vi "Read Monitor Data.vi"(8 "error in (no error)":errorcluster, 11 "Actor Monitor New in":refnum<class "Actor Monitor.lvclass">) -> (0 "error out":errorcluster, 2 "Monitored Actor.lvlib:Monitor Data.lvclass":refnum<class "Monitor Data.lvclass">, 3 "Actor Monitor New out":refnum<class "Actor Monitor.lvclass">)   [LabVIEW 2023, in "Monitored Actor.lvlib" / "Actor Monitor.lvclass"]
uses:
  Actor Monitor.lvclass
  Monitor Data/Monitor Data.lvclass
  Actor Monitor.lvclass/Actor Monitor.ctl
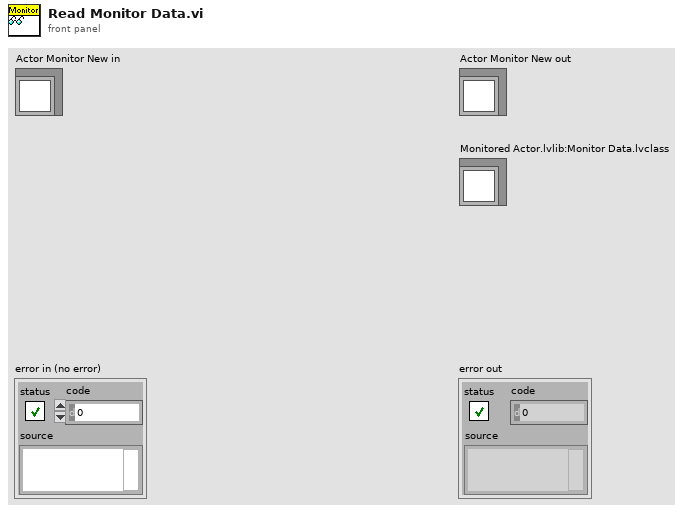
[diagram p1: front panel]
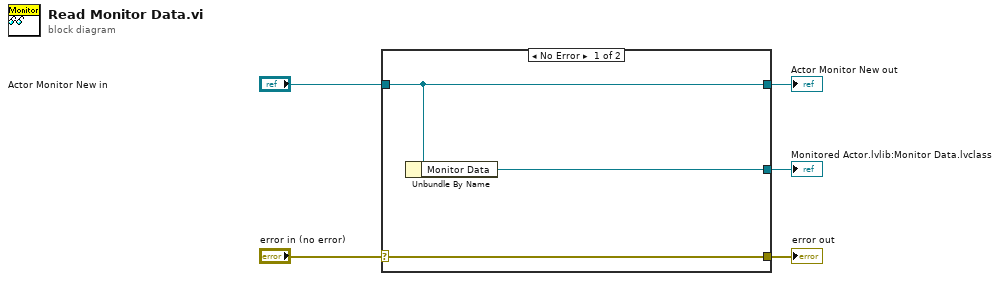
[diagram p0: block diagram]
diagram:
  n1 = case shown="No Error" "error in (no error)" {
    selector: "error in (no error)" -> [w8 w9]
    tunnel: [w8 w9] -> w4
    tunnel: [w7 w10] -> w2
    tunnel: "Actor Monitor New in" -> [w7 w10]
    tunnel: [w6 _] -> w1
    frame No Error {
      n2 = Unbundle By Name(w7) -> ("Monitor Data"=w6:refnum<class "Monitor Data.lvclass">)
    }
    frame Error {
    }
  }
  "error out" <- w4
  "Actor Monitor New out" <- w2
  "Monitored Actor.lvlib:Monitor Data.lvclass" <- w1
